vi "Arc Line Profile.vi"() -> ()   [LabVIEW 2020]
doc: "An example on creating arc line profiles and edge detection in images.\nThis is done in several steps in order for developers to implement custom deviations on the profile and edge detection algorithms."
uses:
  <vilib>/Natan Biesmans/G2CPU GPU and CPU HPC Toolkit/G2CPU Libraries/Arrays/1DArray/binary/1D Array binary.lvclass
  C:/Program Files/National Instruments/LabVIEW 2025/vi.lib/Natan Biesmans/G2CPU GPU and CPU HPC Toolkit/G2CPU Libraries/Arrays/Array/Array Prototype.lvclass
  <vilib>/Natan Biesmans/G2CPU GPU and CPU HPC Toolkit/G2CPU Libraries/Arrays/1DArray/s32/1D Array s32.lvclass
  <vilib>/Natan Biesmans/G2CPU GPU and CPU HPC Toolkit/G2CPU Libraries/Arrays/1DArray/f32/1D Array f32.lvclass
  <vilib>/Natan Biesmans/G2CPU GPU and CPU HPC Toolkit/G2CPU Libraries/Arrays/Array/Array Prototype.lvclass/Array Prototype.ctl
  5f3c4107-8e42-45fc-81f1-860c70d26020.vi
  fa85e424-7d96-4f01-b21a-70d88b3e1ec1.vi
  7bea8c03-5bc2-4de0-b37e-029de35a19e3.vi
  2cd8d775-d0fd-4d24-8ce2-33cbb65880a9.vi
  fbe607f5-0d25-423d-a898-02071c13ba26.vi
  e4f886df-2c09-4170-9ca1-91b4fd3229b7.vi
  95683e00-220f-467d-9aec-fdfa3598d5e1.vi
  3e861b6c-8be5-4daf-94ca-62d312676a27.vi
  6c50b196-f135-46cd-a2a9-1dc6ef1a65d9.vi
  a8ab891f-7333-41a6-9969-d30185546286.vi
  88f05792-a7a0-476a-bf13-f380983a1a42.vi
  c15e7350-ca6b-4d44-b865-c09765c30aed.vi
  e2ff678f-69f2-4586-99d8-fc27b0f69b78.vi
  e09e9b84-bf55-42dc-bfba-0cefc8548f7d.vi
  9a3ae744-4653-4e5b-88f0-64f4fb65b1a5.vi
  c2f5ce90-d43c-444a-91c3-2be840f008e6.vi
  be3aeb34-0b44-4db0-89e6-a017cd8bb556.vi
  <vilib>/Natan Biesmans/G2CPU GPU and CPU HPC Toolkit/G2CPU Libraries/Arrays/SubVI/Array Sizes to Dim Cluster.vi
  5f3c4107-8e42-45fc-81f1-860c70d26020.vi/3a9a0f39-20d0-42ec-98d3-19db30a3fafd.vi
  <vilib>/Natan Biesmans/G2CPU GPU and CPU HPC Toolkit/ArrayFire Driver/VIs/Run as Multi Device.vi
  <vilib>/Natan Biesmans/G2CPU GPU and CPU HPC Toolkit/G2CPU Libraries/Runtime Licensing/G2CPU License Check.vi
  fa85e424-7d96-4f01-b21a-70d88b3e1ec1.vi/3a9a0f39-20d0-42ec-98d3-19db30a3fafd.vi
  7bea8c03-5bc2-4de0-b37e-029de35a19e3.vi/3a9a0f39-20d0-42ec-98d3-19db30a3fafd.vi
  2cd8d775-d0fd-4d24-8ce2-33cbb65880a9.vi/3a9a0f39-20d0-42ec-98d3-19db30a3fafd.vi
  fbe607f5-0d25-423d-a898-02071c13ba26.vi/3a9a0f39-20d0-42ec-98d3-19db30a3fafd.vi
  e4f886df-2c09-4170-9ca1-91b4fd3229b7.vi/3a9a0f39-20d0-42ec-98d3-19db30a3fafd.vi
  95683e00-220f-467d-9aec-fdfa3598d5e1.vi/3a9a0f39-20d0-42ec-98d3-19db30a3fafd.vi
  3e861b6c-8be5-4daf-94ca-62d312676a27.vi/3a9a0f39-20d0-42ec-98d3-19db30a3fafd.vi
  6c50b196-f135-46cd-a2a9-1dc6ef1a65d9.vi/3a9a0f39-20d0-42ec-98d3-19db30a3fafd.vi
  a8ab891f-7333-41a6-9969-d30185546286.vi/ef94ed2d-c4e6-48dc-8bdb-249d71a97973.vi
  <vilib>/Natan Biesmans/G2CPU GPU and CPU HPC Toolkit/G2CPU Libraries/Arrays/Array/G2CPU Get Array Pointer.vi
  88f05792-a7a0-476a-bf13-f380983a1a42.vi/ef94ed2d-c4e6-48dc-8bdb-249d71a97973.vi
  c15e7350-ca6b-4d44-b865-c09765c30aed.vi/ef94ed2d-c4e6-48dc-8bdb-249d71a97973.vi
  e2ff678f-69f2-4586-99d8-fc27b0f69b78.vi/ef94ed2d-c4e6-48dc-8bdb-249d71a97973.vi
  e09e9b84-bf55-42dc-bfba-0cefc8548f7d.vi/ef94ed2d-c4e6-48dc-8bdb-249d71a97973.vi
  9a3ae744-4653-4e5b-88f0-64f4fb65b1a5.vi/ef94ed2d-c4e6-48dc-8bdb-249d71a97973.vi
  c2f5ce90-d43c-444a-91c3-2be840f008e6.vi/ef94ed2d-c4e6-48dc-8bdb-249d71a97973.vi
  be3aeb34-0b44-4db0-89e6-a017cd8bb556.vi/ef94ed2d-c4e6-48dc-8bdb-249d71a97973.vi
  <vilib>/Natan Biesmans/G2CPU GPU and CPU HPC Toolkit/G2CPU Libraries/Arrays/2DArray/f32/2D Array f32.lvclass
  <vilib>/Natan Biesmans/G2CPU GPU and CPU HPC Toolkit/G2CPU Libraries/Arrays/1DArray/u32/1D Array u32.lvclass
  <vilib>/Natan Biesmans/G2CPU GPU and CPU HPC Toolkit/G2CPU Libraries/File IO/Images/G2CPU Load 32b Image.vi
  <vilib>/Natan Biesmans/G2CPU GPU and CPU HPC Toolkit/G2CPU Libraries/Arrays/Array/G2CPU Get Data Type.vi
  <vilib>/Natan Biesmans/G2CPU GPU and CPU HPC Toolkit/G2CPU Libraries/Arrays/Array/G2CPU Array Element Count.vi
  <vilib>/Natan Biesmans/G2CPU GPU and CPU HPC Toolkit/ArrayFire Driver/VIs/is scalar.vi
  <vilib>/Natan Biesmans/G2CPU GPU and CPU HPC Toolkit/ArrayFire Driver/VIs/is empty.vi
  <vilib>/Natan Biesmans/G2CPU GPU and CPU HPC Toolkit/ArrayFire Driver/subvi/Error Converter (ErrCode or Status).vi
  <vilib>/Natan Biesmans/G2CPU GPU and CPU HPC Toolkit/G2CPU Libraries/Arrays/SubVI/G2CPU State.vi
  <vilib>/NI License Manager/Open Session.vi
  <vilib>/NI License Manager/Check License Status.vi
  <vilib>/NI License Manager/Check License Status (Single).vi
  <vilib>/NI License Manager/Activate License.vi
  <vilib>/NI License Manager/Activate License (Single).vi
  <vilib>/NI License Manager/Close Session.vi
  <vilib>/Natan Biesmans/G2CPU GPU and CPU HPC Toolkit/G2CPU Libraries/Arrays/Array/G2CPU Set Array Pointer.vi
  <vilib>/Natan Biesmans/G2CPU GPU and CPU HPC Toolkit/G2CPU Libraries/Arrays/DataTypes/f32/f32.lvclass
  <vilib>/Natan Biesmans/G2CPU GPU and CPU HPC Toolkit/G2CPU Libraries/Arrays/2DArray/2D Array Prototype.lvclass
  <vilib>/Natan Biesmans/G2CPU GPU and CPU HPC Toolkit/G2CPU Libraries/Arrays/1DArray/1D Array Prototype.lvclass
  <vilib>/Natan Biesmans/G2CPU GPU and CPU HPC Toolkit/G2CPU Libraries/File IO/G2CPU File IO.lvlib
  G2CPU Line Profile.lvlib
  <vilib>/Natan Biesmans/G2CPU GPU and CPU HPC Toolkit/G2CPU Libraries/Arrays/Array/Array Prototype.lvclass
panel:
  in  "Rising Edge":bool[](array[boolean])=[FALSE, FALSE]
  in  "Stop Angle":sgl[](array[numeric])=[3.0, 5.0] format="%#_g rad"
  in  "Start Angle":sgl[](array[numeric])=[0.0, 2.0] format="%#_g rad"
  in  "Amounts of Lines":i32[](array[numeric])=[8, 20]
  in  "Treshold":i32[](array[numeric])=[70, 50]
  in  "Outer Radius":sgl[](array[numeric])=[100.0, 150.0] format="%#_g px"
  in  "Inner Radius":sgl[](array[numeric])=[10.0, 10.0] format="%#_g px"
  in  "Center Y":sgl[](array[numeric])=[160.0, 340.0] format="%#_g px"
  in  "Center X":sgl[](array[numeric])=[160.0, 440.0] format="%#_g px"
  in  "Image File":path=path "C:/Program Files/ArrayFire/v3/examples/images/bimodal.jpg"
  out "Original Image":sgl[][](graph)
  out "Line Profiles":sgl[][](graph)
  # "Arc Location"
  # "Arc Sizing"
  # "Edge Detection Parameters"
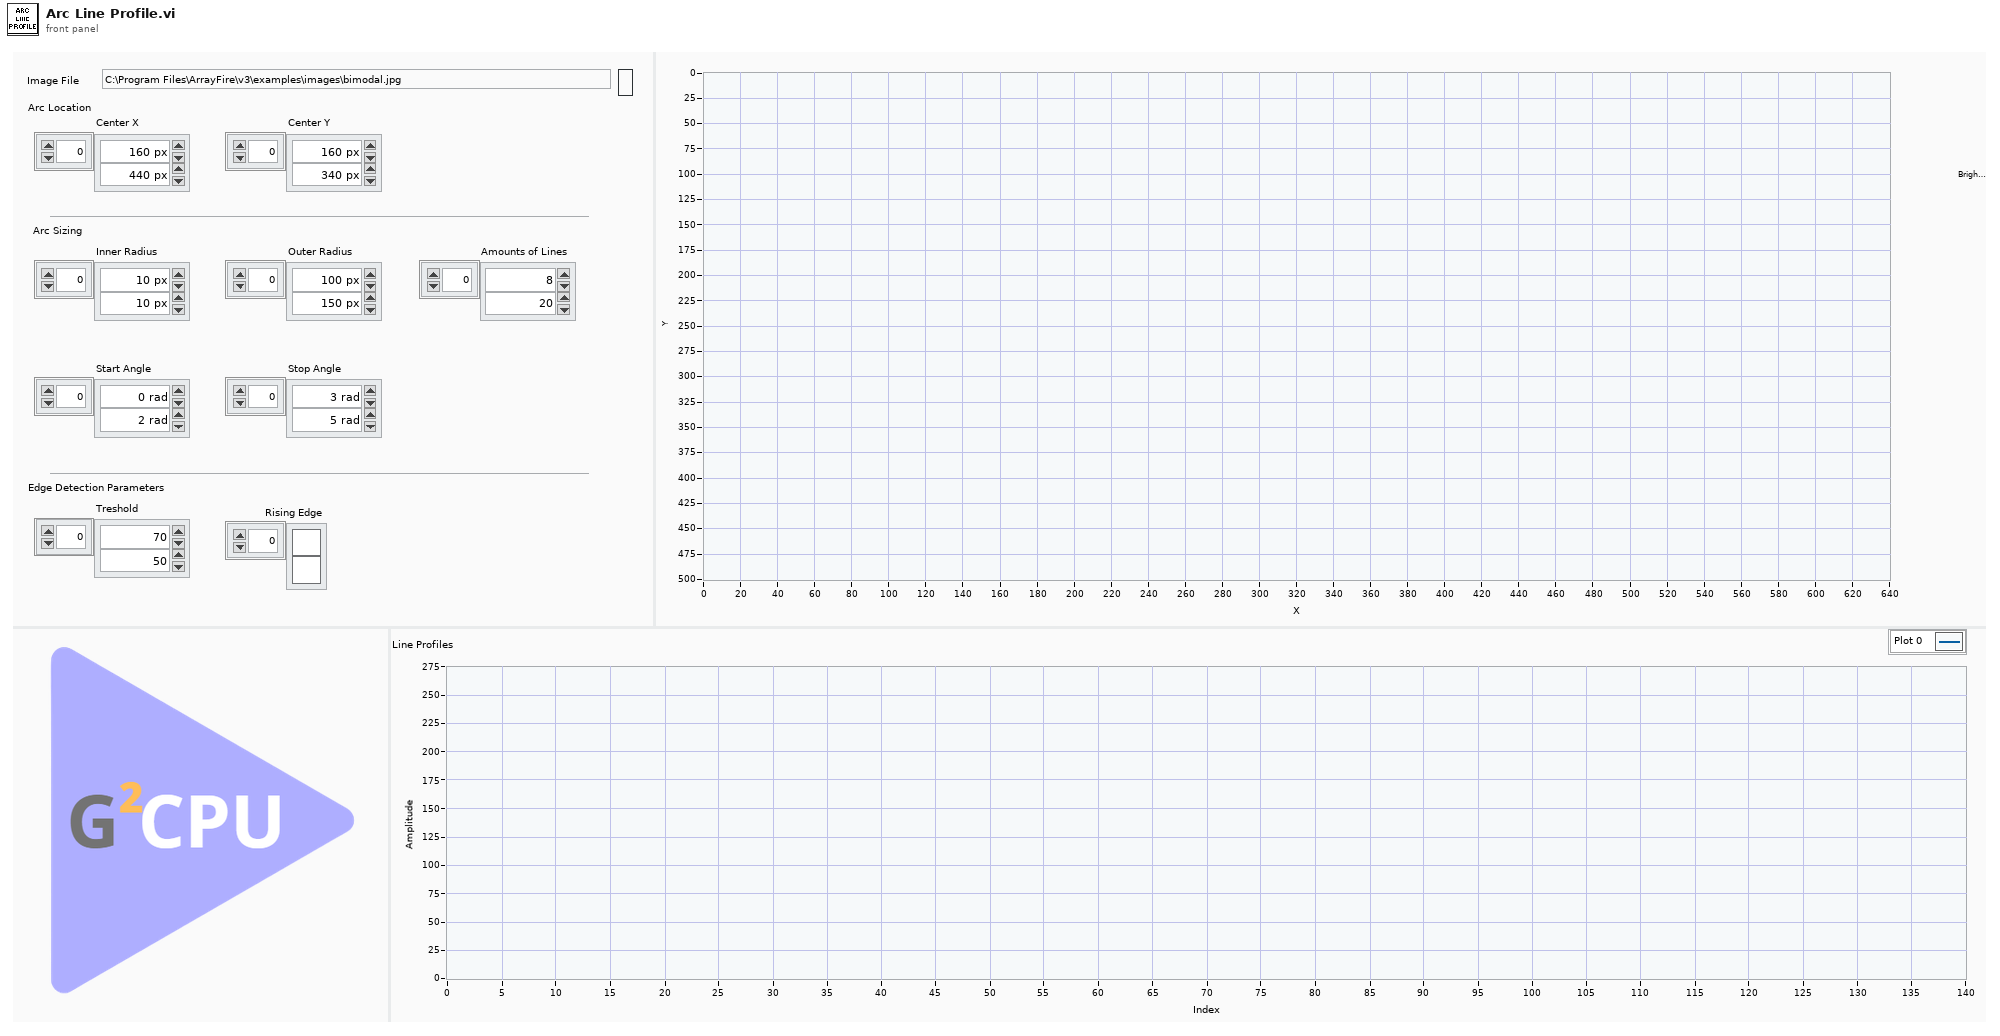
[diagram p1: front panel]
types:
  T1 = cluster{"Center X":refnum<class "1D Array f32.lvclass">, "Center Y":refnum<class "1D Array f32.lvclass">, "Inner Radius":refnum<class "1D Array f32.lvclass">, "Outer Radius":refnum<class "1D Array f32.lvclass">, "Amounts of Lines":refnum<class "1D Array s32.lvclass">, "Stop Angle":refnum<class "1D Array f32.lvclass">, "Start Angle":refnum<class "1D Array f32.lvclass">}
  T2 = cluster{"Rising Edge?":refnum<class "1D Array binary.lvclass">, "Treshold":refnum<class "1D Array s32.lvclass">}
  T3 = cluster{"Auto Release Line Indexers (Enabled)":bool, "Auto Release Keys (Enabled)":bool}
  T4 = cluster{"Points 1 X":refnum<class "1D Array f32.lvclass">, "Points 1 Y":refnum<class "1D Array f32.lvclass">, "Points 2 X":refnum<class "1D Array f32.lvclass">, "Points 2 Y":refnum<class "1D Array f32.lvclass">, "Keys":refnum<class "1D Array u32.lvclass">}
  T5 = cluster{"Line Indexes":refnum<class "2D Array f32.lvclass">, "Keys":refnum<class "2D Array u32.lvclass">, "Index Overflow":u64}
  T6 = cluster{"Line Profiles":refnum<class "2D Array f32.lvclass">, "Keys":refnum<class "2D Array u32.lvclass">}
  T7 = cluster{"X Coordinates":refnum<class "1D Array f32.lvclass">, "Y Coordinates":refnum<class "1D Array f32.lvclass">, "Keys":refnum<class "1D Array u32.lvclass">}
  T8 = cluster{"Name":string, "Color":u32, "Style":u8, "Point Style":u8, "Name Visible":bool, "Allow Drag":bool, "Annotation Mode":u32, "Plot":i32, "Index":i32, "Position":cluster{"X":dbl, "Y":dbl}, "X Scale":u32, "Y Scale":u32, "Show Arrow":bool, "Lock Name":bool, "Plot Area":i32, "Label Offset":cluster{"X":dbl, "Y":dbl}}
  T9 = cluster{"Name":string, "Color":u32, "Style":u8, "Point Style":u8, "Name Visible":bool, "Allow Drag":bool, "Annotation Mode":u32, "Plot":i32, "Index":i32, "Position":cluster{"X":dbl, "Y":dbl}, "X Scale":u32, "Y Scale":u32, "Show Arrow":bool, "Lock Name":bool, "Plot Area":i32, "Label Offset":cluster{"X":dbl, "Y":dbl}}[]
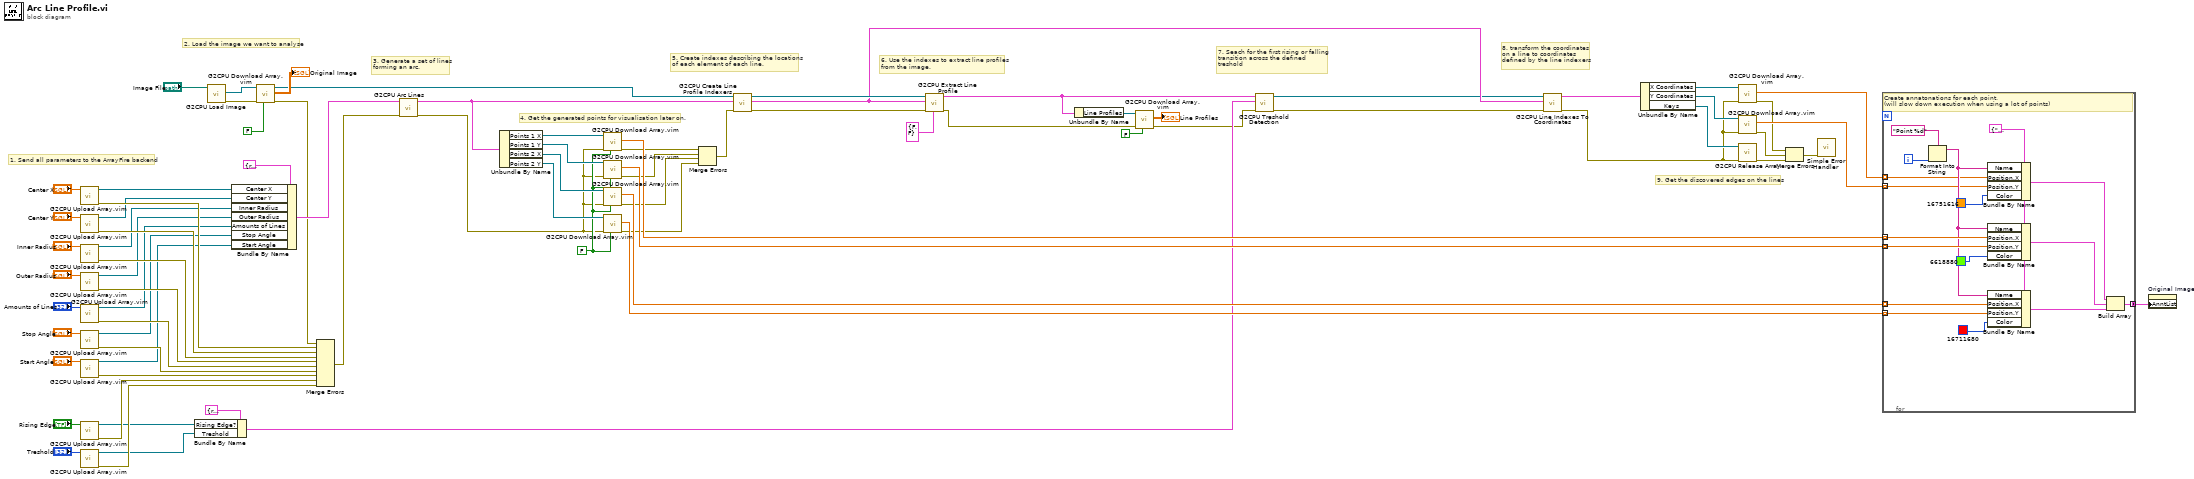
[diagram p0: block diagram]
diagram:
  w53 = FALSE ("Auto Release Array In")
  # "9. Get the discovered edges on the lines"
  # "8. transform the coordinates\non a line to coordinates\ndefined by the line indexers"
  # "7. Seach for the first rising or falling\ntransition across the defined \ntreshold"
  # "6. Use the indexes to extract line profiles \nfrom the image."
  # "5. Create indexes describing the locations\nof each element of each line."
  # "4. Get the generated points for visualisation later on."
  # "3. Generate a set of lines \nforming an arc."
  # "2. Load the image we want to analyse"
  # "1. Send all parameters to the ArrayFire backend"
  n1 = call "G2CPU Upload Array.vim"("Data"="Center X") -> ("error out"=w79:errorcluster, "Array"=w58:refnum<class "1D Array f32.lvclass">)  [unwired: 9 in]
  n2 = call "G2CPU Upload Array.vim"("Data"="Center Y") -> ("error out"=w78:errorcluster, "Array"=w59:refnum<class "1D Array f32.lvclass">)  [unwired: 9 in]
  n3 = call "G2CPU Upload Array.vim"("Data"="Inner Radius") -> ("error out"=w77:errorcluster, "Array"=w60:refnum<class "1D Array f32.lvclass">)  [unwired: 9 in]
  n4 = call "G2CPU Upload Array.vim"("Data"="Outer Radius") -> ("error out"=w76:errorcluster, "Array"=w61:refnum<class "1D Array f32.lvclass">)  [unwired: 9 in]
  n5 = call "G2CPU Upload Array.vim"("Data"="Amounts of Lines") -> ("error out"=w75:errorcluster, "Array"=w62:refnum<class "1D Array s32.lvclass">)  [unwired: 9 in]
  n6 = call "G2CPU Upload Array.vim"("Data"="Stop Angle") -> ("error out"=w74:errorcluster, "Array"=w26:refnum<class "1D Array f32.lvclass">)  [unwired: 9 in]
  n7 = call "G2CPU Upload Array.vim"("Data"="Start Angle") -> ("error out"=w73:errorcluster, "Array"=w29:refnum<class "1D Array f32.lvclass">)  [unwired: 9 in]
  n8 = call "G2CPU Upload Array.vim"("Data"="Rising Edge") -> ("error out"=w72:errorcluster, "Array"=w39:refnum<class "1D Array binary.lvclass">)  [unwired: 9 in]
  n9 = call "G2CPU Upload Array.vim"("Data"="Treshold") -> ("error out"=w71:errorcluster, "Array"=w38:refnum<class "1D Array s32.lvclass">)  [unwired: 9 in]
  n10 = Bundle By Name(cluster=T2 {"Rising Edge?"=refnum, "Treshold"=refnum} ("Treshold Parameters"), "Rising Edge?"=w39, "Treshold"=w38) -> (w40:T2)
  n11 = call-poly <vilib>:"G2CPU Load Image.vi"("Filename"="Image File") -> ("error out"=w69:errorcluster, "Array out"=w70:refnum<class "2D Array f32.lvclass">)  [unwired: 7 in, 2 out]
  n12 = Bundle By Name(cluster=T1 {"Center X"=refnum, "Center Y"=refnum, "Inner Radius"=refnum, "Outer Radius"=refnum, "Amounts of Lines"=refnum, "Stop Angle"=refnum, "Start Angle"=refnum} ("Arc Parameters"), "Center X"=w58, "Center Y"=w59, "Inner Radius"=w60, "Outer Radius"=w61, "Amounts of Lines"=w62, "Stop Angle"=w26, "Start Angle"=w29) -> (w30:T1)
  n13 = call "G2CPU Download Array.vim"("Auto Release Array In"=FALSE, "error in (no error)"=w69, "Array in"=w70) -> ("error out"=w27:errorcluster, "Array Data"=→"Original Image":sgl[][], "Array Out"=w47:refnum<class "2D Array f32.lvclass">)  [unwired: 6 in]
  n14 = Merge Errors(w27, w79, w78, w77, w76, w75, w74, w73, w72, w71) -> (w25:errorcluster)
  n15 = call "G2CPU Arc Lines.vi"("error in (no error)"=w25, "Arc Parameters"=w30) -> ("error out"=w24:errorcluster, "Lines"=w32:T4)  [unwired: 8 in]
  n16 = Unbundle By Name(w32) -> ("Points 1 X"=w54:refnum<class "1D Array f32.lvclass">, "Points 1 Y"=w55:refnum<class "1D Array f32.lvclass">, "Points 2 X"=w56:refnum<class "1D Array f32.lvclass">, "Points 2 Y"=w57:refnum<class "1D Array f32.lvclass">)
  n17 = call "G2CPU Download Array.vim"("Auto Release Array In"=w53, "error in (no error)"=w24, "Array in"=w54) -> ("error out"=w20:errorcluster, "Array Data"=w51:sgl[])  [unwired: 6 in, 1 out]
  n18 = call "G2CPU Download Array.vim"("Auto Release Array In"=w53, "error in (no error)"=w24, "Array in"=w55) -> ("error out"=w21:errorcluster, "Array Data"=w50:sgl[])  [unwired: 6 in, 1 out]
  n19 = call "G2CPU Download Array.vim"("Auto Release Array In"=w53, "error in (no error)"=w24, "Array in"=w56) -> ("error out"=w22:errorcluster, "Array Data"=w49:sgl[])  [unwired: 6 in, 1 out]
  n20 = call "G2CPU Download Array.vim"("Auto Release Array In"=w53, "error in (no error)"=w24, "Array in"=w57) -> ("error out"=w23:errorcluster, "Array Data"=w48:sgl[])  [unwired: 6 in, 1 out]
  n21 = Merge Errors(w20, w21, w22, w23) -> (w19:errorcluster)
  n22 = call "G2CPU Create Line Profile Indexers.vi"("error in (no error)"=w19, "Lines"=w32, "Greyscale Image In"=w47) -> ("error out"=w64:errorcluster, "Line Indexers"=w65:T5, "Greyscale Image Out (inplace)"=w66:refnum<class "2D Array f32.lvclass">)  [unwired: 6 in]
  n23 = call "G2CPU Extract Line Profile.vi"("Auto Release Line Indexers"=T3 {"Auto Release Line Indexers (Enabled)"=FALSE, "Auto Release Keys (Enabled)"=FALSE}, "error in (no error)"=w64, "Line Indexers"=w65, "Greyscale Image In"=w66) -> ("error out"=w13:errorcluster, "Line Profiles Out"=w43:T6)  [unwired: 6 in]
  n24 = Unbundle By Name(w43) -> ("Line Profiles"=w44:refnum<class "2D Array f32.lvclass">)
  n25 = call "G2CPU Download Array.vim"("Auto Release Array In"=FALSE, "error in (no error)"=w13, "Array in"=w44) -> ("error out"=w12:errorcluster, "Array Data"=→"Line Profiles":sgl[][])  [unwired: 6 in, 1 out]
  n26 = call "G2CPU Treshold Detection.vi"("error in (no error)"=w12, "Treshold Parameters"=w40, "Line Profiles"=w43) -> ("error out"=w45:errorcluster, "Edge Indexes out"=w46:refnum<class "1D Array f32.lvclass">)  [unwired: 7 in]
  n27 = call "G2CPU Line Indexes To Coordinates.vi"("error in (no error)"=w45, "Line Indexers"=w65, "Point of Interest on Lines"=w46) -> ("error out"=w18:errorcluster, "Coordinates Out"=w42:T7)  [unwired: 7 in]
  n28 = Unbundle By Name(w42) -> ("X Coordinates"=w34:refnum<class "1D Array f32.lvclass">, "Y Coordinates"=w35:refnum<class "1D Array f32.lvclass">, "Keys"=w33:refnum<class "1D Array u32.lvclass">)
  n29 = call "G2CPU Download Array.vim"("error in (no error)"=w18, "Array in"=w34) -> ("error out"=w17:errorcluster, "Array Data"=w37:sgl[])  [unwired: 7 in, 1 out]
  n30 = call "G2CPU Download Array.vim"("error in (no error)"=w18, "Array in"=w35) -> ("error out"=w16:errorcluster, "Array Data"=w36:sgl[])  [unwired: 7 in, 1 out]
  n31 = call <vilib>:"G2CPU Release Array.vi"("error in (no error)"=w18, "Array in"=w33) -> ("error out"=w15:errorcluster)  [unwired: 9 in]
  n32 = Merge Errors(w17, w16, w15) -> (w10:errorcluster)
  n33 = call <vilib>:"Simple Error Handler.vi"("error in (no error)"=w10) -> ()  [unwired: 4 in, 5 out]
  n34 = for {
    tunnel: [w92] -> w52 mode=concatenating
    tunnel: w51 -> [w89] mode=indexing
    tunnel: w50 -> [w88] mode=indexing
    tunnel: w49 -> [w87] mode=indexing
    tunnel: w48 -> [w86] mode=indexing
    tunnel: w37 -> [w82] mode=indexing
    tunnel: w36 -> [w81] mode=indexing
    i -> [w91]
    w84 = T8 {"Name"="azerty", "Color"=16776960, "Style"=4, "Point Style"=13, "Name Visible"=FALSE, "Allow Drag"=FALSE, "Annotation Mode"=0, "Plot"=-1, "Index"=0, "Position"={"X"=162.8968713789108, "Y"=222.19554030874787}, "X Scale"=0, "Y Scale"=0, "Show Arrow"=FALSE, "Lock Name"=FALSE, "Plot Area"=0, "Label Offset"={"X"=0.0, "Y"=-11.663807890222984}}
    # "Create annatonations for each point.\n(will slow down execution when using a lot of points)"
    n35 = Format Into String(format string="Point %d", w91) -> (resulting string=w83:string)  [unwired: 2 in, 1 out]
    n36 = Bundle By Name(cluster=w84, "Name"=w83, "Position.X"=w82, "Position.Y"=w81, "Color"=u32 16751616) -> (w80:T8)
    n37 = Bundle By Name(cluster=w84, "Name"=w83, "Position.X"=w89, "Position.Y"=w88, "Color"=u32 6618880) -> (w93:T8)
    n38 = Bundle By Name(cluster=w84, "Name"=w83, "Position.X"=w87, "Position.Y"=w86, "Color"=u32 16711680) -> (w94:T8)
    n39 = Build Array(w80, w93, w94) -> (w92:T9)
  }
  n40 = property on="Original Image" class="IntGraph (strict)"("AnntList"=w52) -> ()  [unwired: 2 in, 2 out]
